vi "ForceBalanceMonitor.vi"() -> ()   [LabVIEW 2017]
uses:
  <vilib>/Analysis/baseanly.llb/Mean (DBL).vi
  <vilib>/Analysis/baseanly.llb/A x Vector.vi
  Globals/mainWTControl.vi
  <vilib>/Utility/file.llb/Write To Spreadsheet File (DBL).vi
  <vilib>/Utility/file.llb/Read From Spreadsheet File (DBL).vi
  <vilib>/Analysis/NI_AALBase.lvlib
panel:
  in  "Sampling Period":dbl
  in  "Sampling Freq.":dbl
  in  "x":bool
  out "Fx                     Fy                     Fz                    Mx                   My                    Mz":dbl[](array[numeric])
  in  "stop":bool
  out "Waveform Chart":dynamicdata(graph)
  out "L2                   S                  D2                  L1                  L3                  D1":dbl[](array[numeric])
  out "Amber Check":bool[](array[boolean])
  out "Amber Check Fail":bool
  out "OMFG Check":bool[](array[boolean])
  out "OMFG Check Fail":bool
  out "Mean Convergence":dbl(graph)
  out "Mean Convergence 2":dbl[][](graph)
  in  "Time Target (s)":dbl=10.0
  in  "Blank Button":bool
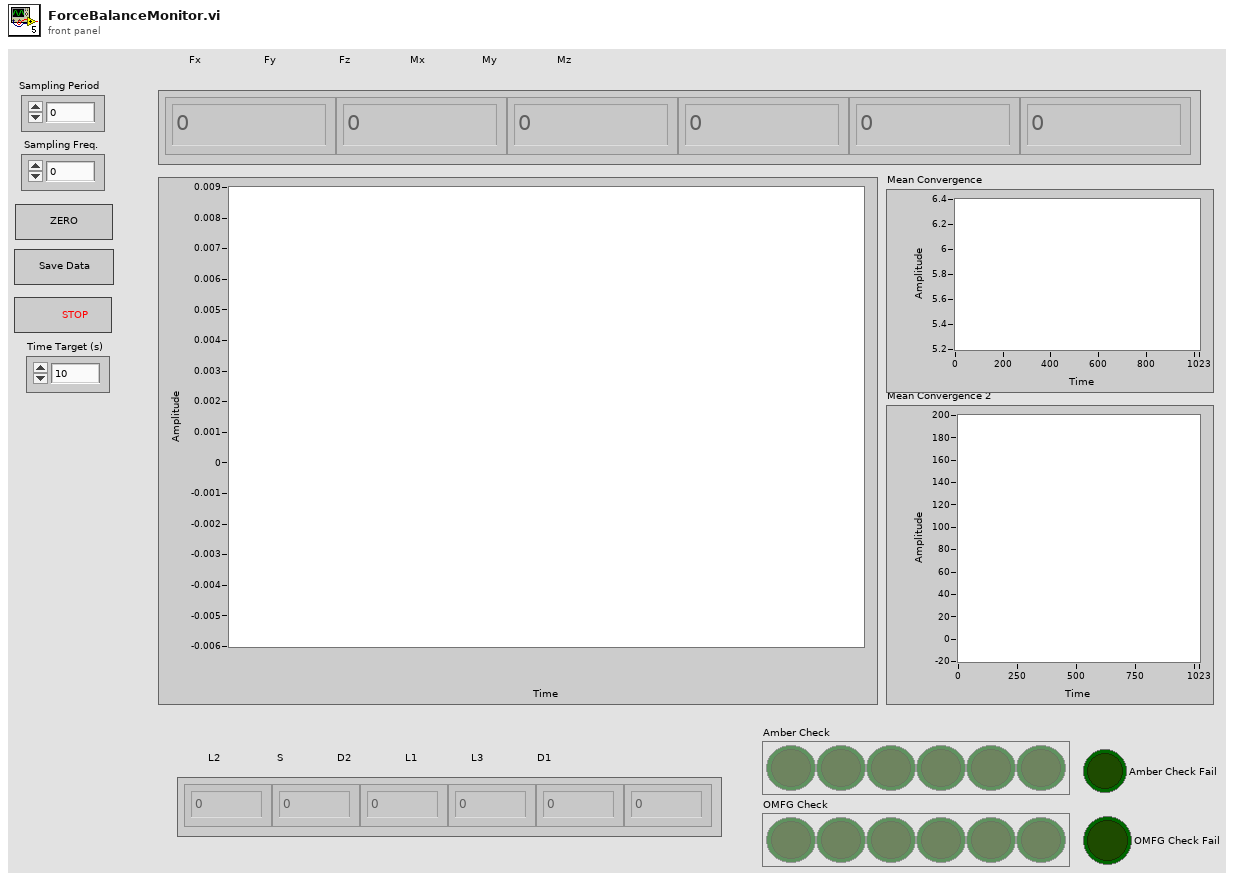
[diagram p1: front panel]
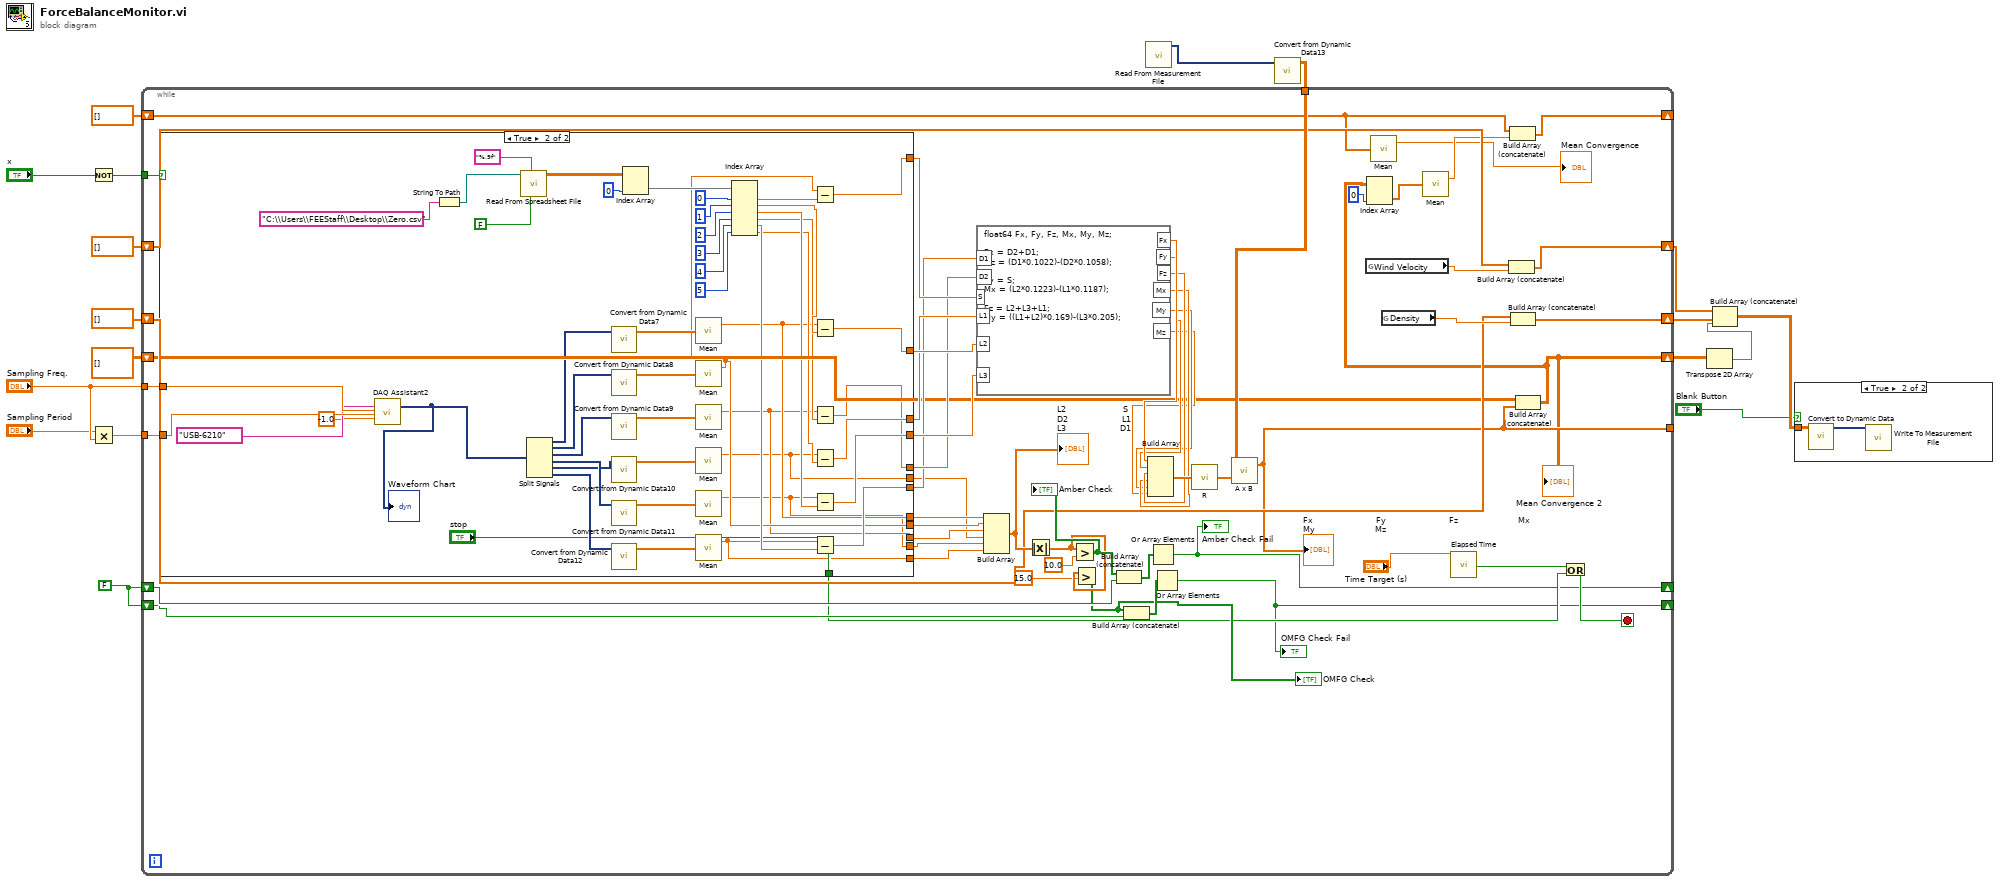
[diagram p0: block diagram]
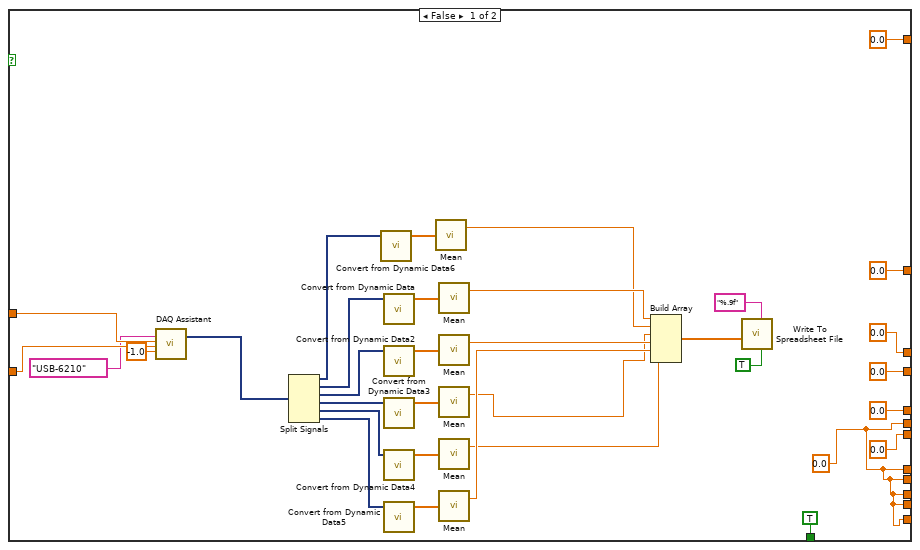
[diagram p3: hidden frame]
diagram:
  w9 = FALSE
  n1 = Not(x="x") -> (.not. x?=w1:bool)
  n2 = Multiply(x="Sampling Period", y="Sampling Freq.") -> (x*y=w5:dbl)
  n3 = call "Read From Measurement File"() -> ("Signals"=w6:dynamicdata)  [unwired: 6 in, 5 out]
  n4 = call "Convert from Dynamic Data13"("Dynamic Data Type"=w6) -> ("Array"=w7:dbl[][])  [unwired: 3 in]
  n5 = while {
    tunnel: w1 -> [w73]
    tunnel: "Sampling Freq." -> [w72]
    tunnel: w5 -> [w71]
    tunnel: [w30] -> _
    tunnel: w7 -> [w70]
    shift-right: [w19] -> _
    shift-left: w9 -> [w47]
    shift-right: [w20] -> _
    shift-left: w9 -> [w42]
    shift-right: [w38] -> w14
    shift-left: dbl[] [] -> [w37]
    shift-right: [w35] -> w12
    shift-left: dbl[] [] -> [w34]
    shift-right: [w25] -> w16
    shift-left: dbl[][] [] -> [w27]
    shift-right: [w26] -> _
    shift-left: dbl[] [] -> [w23]
    stop <- w32 stop-if-true
    n6 = case shown="True" w73 {
      tunnel: [0.0 w122] -> w63
      tunnel: [0.0 w121] -> w62
      tunnel: [0.0 w141] -> w66
      tunnel: [0.0 w140] -> w65
      tunnel: [0.0 w142] -> w64
      tunnel: [0.0 w143] -> w67
      tunnel: w72 -> [w107 w156]
      tunnel: w71 -> [w106 w155]
      tunnel: [TRUE ("stop") "stop"] -> w33
      tunnel: [w74 w113] -> w55
      tunnel: [w74 w112] -> w54
      tunnel: [w74 w111] -> w53
      tunnel: [w74 w110] -> w52
      tunnel: [w74 w109] -> w51
      tunnel: [w74 w108] -> w50
      frame False {
        w74 = 0.0
        n7 = call "DAQ Assistant"("rate"=w107, "number of samples"=w106, "timeout (s)"=-1.0, "device name"=tag "USB-6210") -> ("data"=w93:dynamicdata)  [unwired: 13 in, 2 out]
        n8 = Split Signals(w93) -> (w81:dynamicdata, w92:dynamicdata, w90:dynamicdata, w88:dynamicdata, w86:dynamicdata, w84:dynamicdata)  [unwired: 6 in]
        n9 = call "Convert from Dynamic Data6"("Dynamic Data Type"=w81) -> ("Array"=w77:dbl[])  [unwired: 3 in]
        n10 = call "Convert from Dynamic Data"("Dynamic Data Type"=w92) -> ("Array"=w91:dbl[])  [unwired: 3 in]
        n11 = call "Convert from Dynamic Data2"("Dynamic Data Type"=w90) -> ("Array"=w89:dbl[])  [unwired: 3 in]
        n12 = call "Convert from Dynamic Data3"("Dynamic Data Type"=w88) -> ("Array"=w87:dbl[])  [unwired: 3 in]
        n13 = call "Convert from Dynamic Data4"("Dynamic Data Type"=w86) -> ("Array"=w85:dbl[])  [unwired: 3 in]
        n14 = call "Convert from Dynamic Data5"("Dynamic Data Type"=w84) -> ("Array"=w83:dbl[])  [unwired: 3 in]
        n15 = call-poly <vilib>:"Mean.vi"("X"=w77) -> ("mean"=w95:dbl)  [unwired: 1 out]
        n16 = call-poly <vilib>:"Mean.vi"("X"=w91) -> ("mean"=w98:dbl)  [unwired: 1 out]
        n17 = call-poly <vilib>:"Mean.vi"("X"=w89) -> ("mean"=w97:dbl)  [unwired: 1 out]
        n18 = call-poly <vilib>:"Mean.vi"("X"=w87) -> ("mean"=w78:dbl)  [unwired: 1 out]
        n19 = call-poly <vilib>:"Mean.vi"("X"=w85) -> ("mean"=w76:dbl)  [unwired: 1 out]
        n20 = call-poly <vilib>:"Mean.vi"("X"=w83) -> ("mean"=w96:dbl)  [unwired: 1 out]
        n21 = Build Array(w98, w95, w78, w97, w96, w76) -> (w94:dbl[])
        n22 = call-poly <vilib>:"Write To Spreadsheet File.vi"("transpose? (no:F)"=TRUE, "format (%.3f)"="%.9f", "1D data"=w94) -> ()  [unwired: 5 in, 1 out]
      }
      frame True {
        n23 = call "DAQ Assistant2"("rate"=w156, "number of samples"=w155, "timeout (s)"=-1.0, "device name"=tag "USB-6210") -> ("data"=w114:dynamicdata)  [unwired: 12 in, 3 out]
        "Waveform Chart" <- w114
        n24 = String To Path(string="C:\\Users\\FEEStaff\\Desktop\\Zero.csv" ("format (%.3f)")) -> (path=w123:path)
        n25 = call-poly <vilib>:"Read From Spreadsheet File.vi"("transpose (no:F)"=FALSE, "format (%.3f)"="%.9f", "file path (dialog if empty)"=w123) -> ("all rows"=w146:dbl[][])  [unwired: 4 in, 4 out]
        n26 = Split Signals(w114) -> (w130:dynamicdata, w136:dynamicdata, w134:dynamicdata, w117:dynamicdata, w116:dynamicdata, w131:dynamicdata)  [unwired: 6 in]
        n27 = call "Convert from Dynamic Data7"("Dynamic Data Type"=w130) -> ("Array"=w137:dbl[])  [unwired: 3 in]
        n28 = call "Convert from Dynamic Data8"("Dynamic Data Type"=w136) -> ("Array"=w135:dbl[])  [unwired: 3 in]
        n29 = call "Convert from Dynamic Data9"("Dynamic Data Type"=w134) -> ("Array"=w119:dbl[])  [unwired: 3 in]
        n30 = call "Convert from Dynamic Data10"("Dynamic Data Type"=w116) -> ("Array"=w133:dbl[])  [unwired: 3 in]
        n31 = call "Convert from Dynamic Data11"("Dynamic Data Type"=w117) -> ("Array"=w132:dbl[])  [unwired: 3 in]
        n32 = call "Convert from Dynamic Data12"("Dynamic Data Type"=w131) -> ("Array"=w120:dbl[])  [unwired: 3 in]
        n33 = Index Array(array=w146, index (col)=0 ("disabled index (col)")) -> (element=w144:dbl[])  [unwired: 1 in]
        n34 = call-poly <vilib>:"Mean.vi"("X"=w137) -> ("mean"=w113:dbl)  [unwired: 1 out]
        n35 = call-poly <vilib>:"Mean.vi"("X"=w135) -> ("mean"=w112:dbl)  [unwired: 1 out]
        n36 = call-poly <vilib>:"Mean.vi"("X"=w119) -> ("mean"=w111:dbl)  [unwired: 1 out]
        n37 = call-poly <vilib>:"Mean.vi"("X"=w133) -> ("mean"=w110:dbl)  [unwired: 1 out]
        n38 = call-poly <vilib>:"Mean.vi"("X"=w132) -> ("mean"=w109:dbl)  [unwired: 1 out]
        n39 = call-poly <vilib>:"Mean.vi"("X"=w120) -> ("mean"=w108:dbl)  [unwired: 1 out]
        n40 = Index Array(array=w144, index #1=0 ("index (row)"), index #2=1 ("index (row)"), index #3=2 ("index (row)"), index #4=3 ("index (row)"), index #5=4 ("index (row)"), index #6=5 ("index (row)")) -> (element #1=w129:dbl, element #2=w128:dbl, element #3=w127:dbl, element #4=w126:dbl, element #5=w125:dbl, element #6=w118:dbl)
        n41 = Subtract(x=w112, y=w129) -> (x-y=w143:dbl)
        n42 = Subtract(x=w113, y=w128) -> (x-y=w141:dbl)
        n43 = Subtract(x=w111, y=w126) -> (x-y=w122:dbl)
        n44 = Subtract(x=w110, y=w118) -> (x-y=w140:dbl)
        n45 = Subtract(x=w109, y=w127) -> (x-y=w142:dbl)
        n46 = Subtract(x=w108, y=w125) -> (x-y=w121:dbl)
      }
    }
    n47 = formula code="float64 Fx, Fy, Fz, Mx, My, Mz;\n\nFx = D2+D1;\nMz = (D1*0.1022)-(D2*0.1058);\n\nFy = S;\nMx = (L2*0.1223)-(L1*0.1187);\n\nFz = L2+L3+L1;\nMy = ((L1+L2)*0.169)-(L3*0.205);"("D1"=w62, "D2"=w63, "S"=w67, "L1"=w65, "L2"=w66, "L3"=w64) -> ("Fx"=w61:dbl, "Fy"=w60:dbl, "Fz"=w59:dbl, "Mx"=w58:dbl, "My"=w57:dbl, "Mz"=w56:dbl)
    n48 = Build Array(w55, w54, w53, w52, w51, w50) -> (w49:dbl[])
    "L2                   S                  D2                  L1                  L3                  D1" <- w49
    n49 = Absolute Value(x=w49) -> (abs(x)=w44:dbl[])
    n50 = Greater?(x=w44, y=10.0 ("Numeric")) -> (0:w45:bool[])
    "Amber Check" <- w45
    n51 = Greater?(x=w44, y=15.0) -> (0:w40:bool[])
    "OMFG Check" <- w40
    n52 = Build Array (concatenate)(w45, w47) -> (w46:bool[])
    n53 = Build Array (concatenate)(w40, w42) -> (w41:bool[])
    n54 = Build Array(w61, w60, w59, w58, w57, w56) -> (w68:dbl[])
    n55 = Or Array Elements(Boolean array=w46) -> (logical OR=w19:bool)
    "Amber Check Fail" <- w19
    n56 = Or Array Elements(Boolean array=w41) -> (logical OR=w20:bool)
    "OMFG Check Fail" <- w20
    n57 = call "R.vi"("1x6"=w68) -> ("27x1"=w69:dbl[])
    n58 = call-poly <vilib>:"A x B.vi"("Vector"=w69, "A"=w70) -> ("A x Vector"=w30:dbl[])  [unwired: 1 out]
    "Fx                     Fy                     Fz                    Mx                   My                    Mz" <- w30
    n59 = global read "mainWTControl.vi" "Wind Velocity"() -> (w39:dbl)
    n60 = call-poly <vilib>:"Mean.vi"("X"=w23) -> ("mean"=→"Mean Convergence":dbl)  [unwired: 1 out]
    n61 = global read "mainWTControl.vi" "Density"() -> (w36:dbl)
    n62 = call "Elapsed Time"("Time Target (s)"="Time Target (s)") -> ("Time has Elapsed"=w31:bool)  [unwired: 11 in, 7 out]
    n63 = Build Array (concatenate)(w37, w39) -> (w38:dbl[])
    n64 = Build Array (concatenate)(w34, w36) -> (w35:dbl[])
    n65 = Build Array (concatenate)(w27, w30) -> (w25:dbl[][])
    "Mean Convergence 2" <- w25
    n66 = Index Array(array=w25, index (col)=0 ("index")) -> (element=w28:dbl[])  [unwired: 1 in]
    n67 = call-poly <vilib>:"Mean.vi"("X"=w28) -> ("mean"=w24:dbl)  [unwired: 1 out]
    n68 = Build Array (concatenate)(w23, w24) -> (w26:dbl[])
    n69 = Or(x=w31, y=w33) -> (x .or. y?=w32:bool)
  }
  n70 = Transpose 2D Array(2D array=w16) -> (transposed array=w17:dbl[][])
  n71 = Build Array (concatenate)(w14, w12, w17) -> (w18:dbl[][])
  n72 = case shown="True" "Blank Button" {
    tunnel: w18 -> [_ w158]
    frame False {
    }
    frame True {
      n73 = call "Convert to Dynamic Data"("2D Array"=w158) -> ("Dynamic Data Type"=w157:dynamicdata)  [unwired: 3 in]
      n74 = call "Write To Measurement File"("Signals"=w157) -> ()  [unwired: 16 in, 3 out]
    }
  }
